vi "SetTextToComboCtrl.vi"(10 "string":string, 11 "ref in":refnum<vi>) -> (3 "ref out":refnum<vi>)   [LabVIEW 2018, in "Library-Ctrl.lvlib"]
uses:
  Library-Ctrl.lvlib
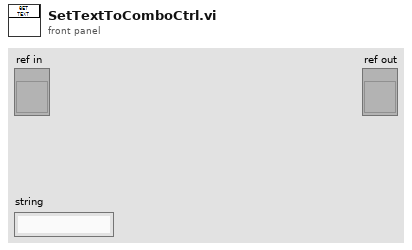
[diagram p1: front panel]
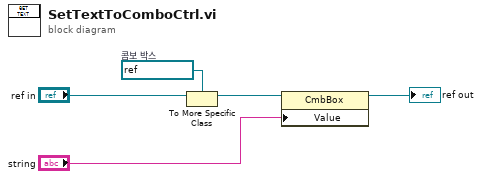
[diagram p0: block diagram]
diagram:
  w3 = refnum<vi> refnum  # 콤보 박스
  n1 = To More Specific Class(target class=w3, reference="ref in") -> (specific class reference=w1:refnum<vi>)  [unwired: 1 in, 1 out]
  n2 = property class="CmbBox"(reference=w1, "Value"="string") -> (reference out=→"ref out":refnum<vi>)  [unwired: 1 in, 1 out]
